vi "mag2db.vi"(1 "Array":dbl[](array[numeric])) -> (0 "x*y":dbl[](array[numeric]))   [LabVIEW 2014]
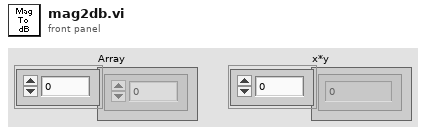
[diagram p1: front panel]
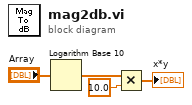
[diagram p0: block diagram]
diagram:
  n1 = Logarithm Base 10(1:"Array") -> (0:w3:dbl[])
  n2 = Multiply(x=w3, y=10.0) -> (x*y=→"x*y":dbl[])
